vi "hasMoved.vi"(1 "read string 2":string="\n") -> (0 "move":bool)   [LabVIEW 2017, in "Monochromator.lvlib"]
doc: "convert wavelength to valtage for DAC"
uses:
  Monochromator.lvlib
panel:
  out "number":i32
  out "move":string
  out "error out":errorcluster
  in  "error in (no error)":errorcluster
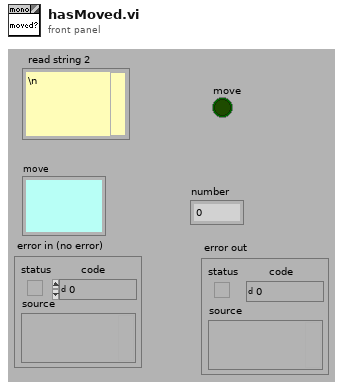
[diagram p1: front panel]
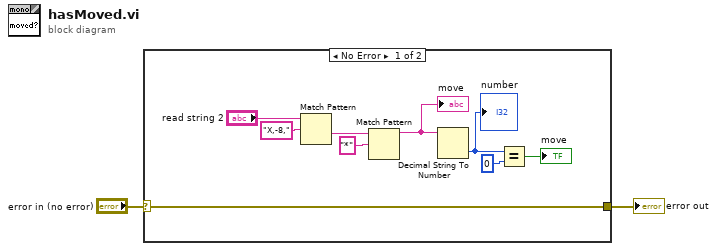
[diagram p0: block diagram]
diagram:
  n1 = case shown="No Error" "error in (no error)" {
    selector: "error in (no error)" -> [w11 w12]
    tunnel: [w11 w12] -> w1
    frame No Error {
      n2 = Match Pattern(string="read string 2", regular expression="X,-8,") -> (after substring=w6:string)  [unwired: 1 in, 3 out]
      n3 = Match Pattern(string=w6, regular expression="*") -> (before substring=w5:string)  [unwired: 1 in, 3 out]
      "move" <- w5
      n4 = Decimal String To Number(string=w5) -> (number=w4:i32)  [unwired: 2 in, 1 out]
      "number" <- w4
      n5 = Equal?(x=w4, y=0) -> (x = y?=→"move":bool)
    }
    frame Error {
    }
  }
  "error out" <- w1
